vi "Complex SVD Decomposition.vi"(9 "SVD option":T2 items=["Thin", "Full"], 10 "singular values only?":bool, 11 "A":T1) -> (0 "error":i32, 1 "Matrix V":T1, 2 "Matrix S":T1, 3 "Matrix U":T1, 5 "Vector S":dbl[](array[numeric]))   [LabVIEW 2010, in "NI_AALPro.lvlib"]
doc: "Computes the singular value decomposition (SVD) of the m x n matrix <B>A</B>. Wire data to the <B>A</B> input to determine the polymorphic instance to use or manually select the instance."
uses:
  NI_AALPro.lvlib
  ComplexMatrix.ctl
  SVD Option.ctl
  Create Special Real Matrix.vi
  lvanlys.dll
  NI_Matrix.lvlib
panel:
  # "Complex SVD Decomposition"
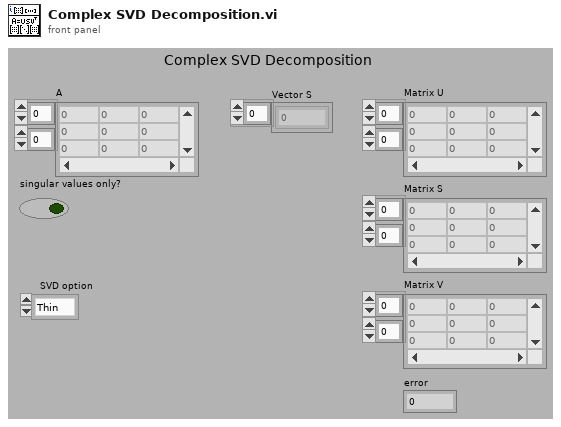
[diagram p1: front panel]
types:
  T1 = typedef "NI_Matrix.lvlib/ComplexMatrix.ctl" = cdb[][]
  T2 = typedef "NI_AALPro.lvlib/SVD Option.ctl" = u16
  T3 = enum32{"Identity", "Diagonal", "Toepliz", "Vandermonde", "Companion"}
  T4 = typedef "NI_Matrix.lvlib/RealMatrix.ctl" = dbl[][]
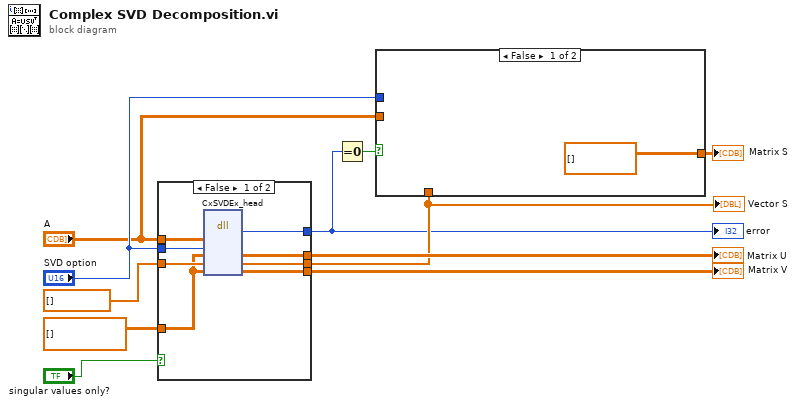
[diagram p0: block diagram]
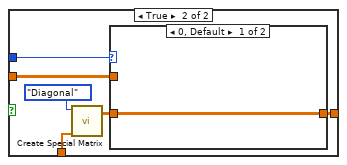
[diagram p2: hidden frame]
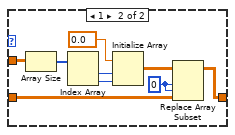
[diagram p3: hidden frame]
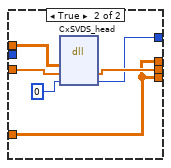
[diagram p4: hidden frame]
diagram:
  n1 = case shown="False" "singular values only?" {
    tunnel: [w19 w21] -> w11
    tunnel: [w18 w21] -> w10
    tunnel: [w17 w20] -> w1
    tunnel: dbl[] [] ("S") -> [w16 w24]
    tunnel: "SVD option" -> [w15 _]
    tunnel: [w14 w22] -> w7
    tunnel: "A" -> [w13 w25]
    tunnel: cdb[][] [] ("S") -> [w12 w21]
    frame False {
      n2 = dll-call lib="C:/Program Files/National Instruments/LabVIEW 2010/resource/lvanlys.*" fn="CxSVDEx_head"("A"=w13, "flag"=w15, "S"=w12, "S"=w16, "S"=w12) -> (w17:i32, "S"=w19:cdb[][], "S"=w14:dbl[], "S"=w18:cdb[][])  [unwired: 5 in, 2 out]
    }
    frame True {
      n3 = dll-call lib="C:/Program Files/National Instruments/LabVIEW 2010/resource/lvanlys.*" fn="CxSVDS_head"("A"=w25, "S"=w24, "input param"=0) -> ("S"=w22:dbl[], "input param"=w20:i32)  [unwired: 5 in, 2 out]
    }
  }
  "Matrix U" <- w11
  "Matrix V" <- w10
  "error" <- w1
  "Vector S" <- w7
  n4 = Equal To 0?(x=w1) -> (x = 0?=w2:bool)
  n5 = case shown="False" w2 {
    tunnel: "SVD option" -> [_ w32]
    tunnel: w7 -> [_ w31]
    tunnel: [T1 [] ("Matrix S") w28] -> w6
    tunnel: "A" -> [_ w27]
    frame False {
    }
    frame True {
      n6 = call-poly "Create Special Matrix.vi"("matrix type"=T3."Diagonal", "Input Vector1"=w31) -> ("Special Matrix"=w29:T4)  [unwired: 3 in, 1 out]
      n7 = case shown="0, Default" w32 {
        tunnel: [w33 w34] -> w28
        tunnel: w29 -> [w33 w35]
        tunnel: w27 -> [_ w39]
        frame 0, Default {
        }
        frame 1 {
          w36 = 0 ("index (row)")
          n8 = Array Size(array=w39) -> (size(s)=w38:i32[])
          n9 = Index Array(array=w38) -> (element #1=w41:i32, element #2=w40:i32)  [unwired: 2 in]
          n10 = Initialize Array(0.0 ("element"), w41, w40) -> (w37:dbl[][])
          n11 = Replace Array Subset(array=w37, new element=w35, index (row)=w36, index (col)=w36) -> (w34:dbl[][])
        }
      }
    }
  }
  "Matrix S" <- w6
